vi "Error Query.vi"(8 "error in (no error)":errorcluster, 11 "VISA resource name":refnum<visa-resource-name>) -> (0 "error out":errorcluster, 1 "Error Message":string, 2 "Error Code":i32[](array[numeric]), 3 "VISA resource name out":refnum<visa-resource-name>)   [LabVIEW 2023, in "Keithley DMM6500 DAQ6500 Series.lvlib"]
doc: "Queries the instrument for any errors in the instrument's error queue. It will continue to read errors until all errors have been read from the instrument. Any errors will be returned in the <B>error out</B> control.\n\n<B>Note:</B>\nThis VI is called automatically by most driver VIs so it is not usually necessary to call this in an application."
uses:
  <instrlib>/Keithley DMM6500 DAQ6500 Series/Keithley DMM6500 DAQ6500 Series.lvlib
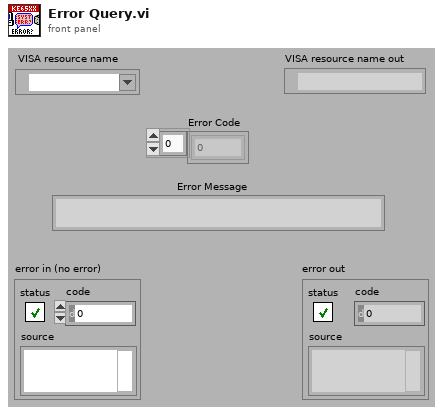
[diagram p1: front panel]
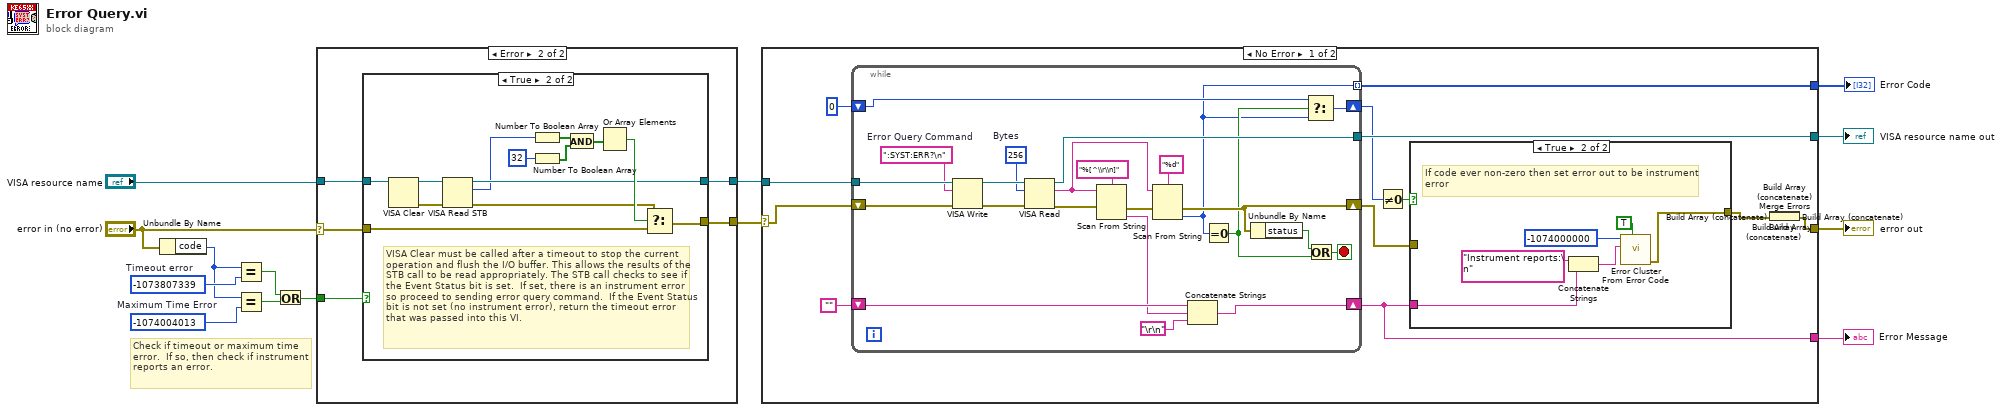
[diagram p0: block diagram]
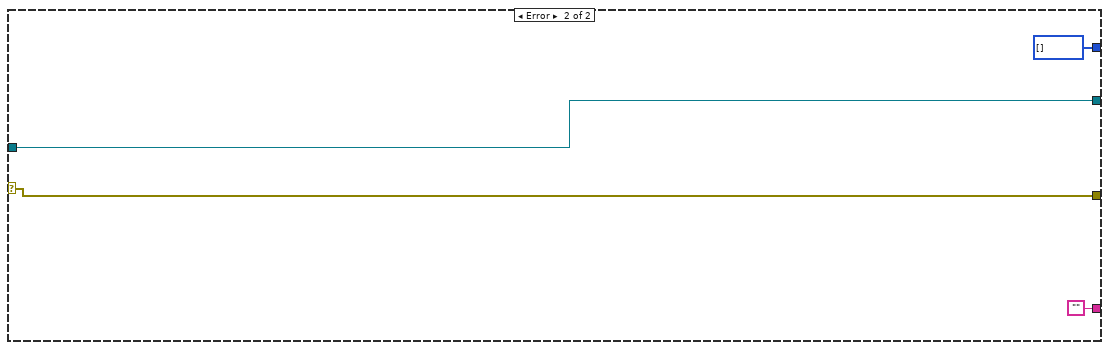
[diagram p5: hidden frame]
diagram:
  w5 = -1074004013  # Maximum Time Error
  w7 = -1073807339  # Timeout error
  # "Check if timeout or maximum time error.  If so, then check if instrument reports an error."
  n1 = Unbundle By Name("error in (no error)") -> ("code"=w6:i32)
  n2 = Equal?(x=w6, y=w7) -> (x = y?=w3:bool)
  n3 = Equal?(x=w6, y=w5) -> (x = y?=w4:bool)
  n4 = Or(x=w3, y=w4) -> (x .or. y?=w2:bool)
  n5 = case shown="Error" "error in (no error)" {
    selector: "error in (no error)" -> [w15 w19]
    tunnel: "VISA resource name" -> [w16 w21]
    tunnel: [w16 w20] -> w9
    tunnel: [w15 w18] -> w10
    tunnel: w2 -> [_ w17]
    frame No Error {
    }
    frame Error {
      n6 = case shown="True" w17 {
        tunnel: w21 -> [w23 w29]
        tunnel: [w23 w26] -> w20
        tunnel: w19 -> [w22 w32]
        tunnel: [w22 w31] -> w18
        frame False {
          # "Error code not a timeout, so best to pass on to user."
        }
        frame True {
          # "VISA Clear must be called after a timeout to stop the current operation and flush the I/O buffer. This allows the results of the  STB call to be read appropriately. The STB call checks to see if the Event Status bit is set.  If set, there is an instrument error so proceed to sending error query command.  If the Event Status bit is not set (no instrument error), return the timeout error that was passed into this VI."
          n7 = VISA Clear(VISA resource name=w29) -> (VISA resource name out=w28:refnum<visa-resource-name>, error out=w27:errorcluster)  [unwired: 1 in]
          n8 = VISA Read STB(8:w27, 11:w28) -> (0:w25:errorcluster, 2:w24:u16, 3:w26:refnum<visa-resource-name>)
          n9 = Number To Boolean Array(number=w24) -> (Boolean array=w33:bool[])
          n10 = Number To Boolean Array(number=32) -> (Boolean array=w35:bool[])
          n11 = And(x=w33, y=w35) -> (x .and. y?=w34:bool[])
          n12 = Or Array Elements(Boolean array=w34) -> (logical OR=w30:bool)
          n13 = Select(t=w25, s=w30, f=w32) -> (s? t:f=w31:errorcluster)
        }
      }
    }
  }
  n14 = case shown="No Error" w10 {
    selector: w10 -> [w42 w84]
    tunnel: [w53 w87] -> w14
    tunnel: w9 -> [w52 w87]
    tunnel: [w50 w84] -> w13
    tunnel: [w45 ""] -> w12
    tunnel: [w44 i32[] []] -> w11
    frame No Error {
      n15 = while {
        tunnel: [w83] -> w53
        tunnel: w52 -> [w82]
        shift-right: [w70] -> w45
        shift-left: "" -> [w73]
        shift-right: [w68] -> w46
        shift-left: 0 -> [w69]
        shift-right: [w66] -> w43
        shift-left: w42 -> [w67]
        tunnel: [w61] -> w44 mode=indexing
        stop <- w76 stop-if-true
        w80 = u32 256  # Bytes
        w78 = ":SYST:ERR?\n"  # Error Query Command
        n16 = VISA Write(VISA resource name=w82, write buffer=w78, error in (no error)=w67) -> (VISA resource name out=w81:refnum<visa-resource-name>, error out=w79:errorcluster)  [unwired: 1 out]
        n17 = VISA Read(VISA resource name=w81, byte count=w80, error in (no error)=w79) -> (VISA resource name out=w83:refnum<visa-resource-name>, read buffer=w74:string, error out=w65:errorcluster)  [unwired: 1 out]
        n18 = Scan From String(format string="%[^\\r\\n]", input string=w74, error in=w65) -> (error out=w64:errorcluster, output 1=w71:string)  [unwired: 2 in, 2 out]
        n19 = Scan From String(format string="%d", input string=w74, error in=w64) -> (error out=w66:errorcluster, output 1=w61:i32)  [unwired: 2 in, 2 out]
        n20 = Concatenate Strings(w73, w71, "\r\n") -> (w70:string)
        n21 = Equal To 0?(x=w61) -> (x = 0?=w62:bool)
        n22 = Unbundle By Name(w66) -> ("status"=w63:bool)
        n23 = Select(t=w69, s=w62, f=w61) -> (s? t:f=w68:i32)
        n24 = Or(x=w63, y=w62) -> (x .or. y?=w76:bool)
      }
      n25 = Not Equal To 0?(x=w46) -> (x != 0?=w48:bool)
      n26 = case shown="True" w48 {
        tunnel: w45 -> [_ w59]
        tunnel: [w54 w55] -> w47
        tunnel: w43 -> [w54 _]
        frame False {
        }
        frame True {
          # "If code ever non-zero then set error out to be instrument error"
          n27 = Concatenate Strings("Instrument reports:\n" ("Source"), w59) -> (w56:string)
          n28 = call <vilib>:"Error Cluster From Error Code.vi"("show call chain? (False)"=TRUE, "error message (\"\")"=w56, "error code (0)"=-1074000000 ("Code")) -> ("error out"=w55:errorcluster)  [unwired: 6 in]
        }
      }
      n29 = Build Array(w47) -> (w41:errorcluster[])
      n30 = Build Array (concatenate)(w41) -> (w40:errorcluster[])
      n31 = Build Array (concatenate)(w40) -> (w39:errorcluster[])
      n32 = Build Array (concatenate)(w39) -> (w38:errorcluster[])
      n33 = Build Array (concatenate)(w38) -> (w37:errorcluster[])
      n34 = Merge Errors(w37) -> (w50:errorcluster)
    }
    frame Error {
    }
  }
  "VISA resource name out" <- w14
  "error out" <- w13
  "Error Message" <- w12
  "Error Code" <- w11
